vi "myRIO v1.0 Build MUX Configuration DIO.vi"(11 "DIO Channel List":T4) -> (2 "Configuration Bitmask Array":bool[][](array[boolean]), 3 "Channel Reservation List":T1)   [LabVIEW 2021]
uses:
  <vilib>/myRIO/Common/Instrument Driver Framework/myRIO v1.0/DIO/typedefs/DIO Channels List.ctl
  <vilib>/myRIO/Common/Instrument Driver Framework/myRIO v1.0/DIO/typedefs/DIO Channels Enum.ctl
  <vilib>/myRIO/Common/Instrument Driver Framework/myRIO v1.0/Resource Manager/typedefs/myRIO v1.0 Channel Reservation List.ctl
  <vilib>/myRIO/Common/Instrument Driver Framework/myRIO v1.0/Resource Manager/typedefs/myRIO v1.0 Channel Reservation Info.ctl
  <vilib>/myRIO/Common/Instrument Driver Framework/myRIO v1.0/Resource Manager/typedefs/myRIO v1.0 Connector List.ctl
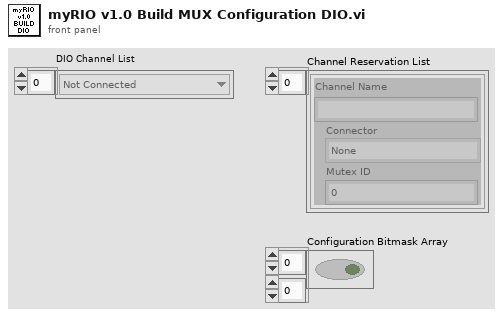
[diagram p1: front panel]
types:
  T1 = typedef "myRIO v1.0 Channel Reservation List.ctl" = T2[]
  T2 = typedef "myRIO v1.0 Channel Reservation Info.ctl" = cluster{"Channel Name":string, "Connector":T3, "Mutex ID":i32}
  T3 = typedef "myRIO v1.0 Connector List.ctl" = enum32{"None", "ConnectorA", "ConnectorB", "ConnectorC"}
  T4 = typedef "DIO Channels List.ctl" = T5[]
  T5 = typedef "DIO Channels Enum.ctl" = enum16{"Not Connected", "C/DIO0", "C/DIO1", "C/DIO2", "C/DIO3", "C/DIO4", "C/DIO5", "C/DIO6", "C/DIO7", "A/DIO0", "A/DIO1", "A/DIO2", "A/DIO3", "A/DIO4", "A/DIO5", "A/DIO6", "A/DIO7", "A/DIO8", "A/DIO9", "A/DIO10", "A/DIO11", "A/DIO12", "A/DIO13", "A/DIO14", "A/DIO15", "A/DIO16", "A/DIO17", "A/DIO18", "A/DIO19", "B/DIO0", "B/DIO1", "B/DIO2", "B/DIO3", "B/DIO4", "B/DIO5", "B/DIO6", "B/DIO7", "B/DIO8", "B/DIO9", "B/DIO10", "B/DIO11", "B/DIO12", "B/DIO13", "B/DIO14", "B/DIO15", "B/DIO16", "B/DIO17", "B/DIO18", "B/DIO19", "LED0", "LED1", "LED2", "LED3", "Button0", "DIO/DIO0", "DIO/DIO1", "DIO/DIO2", "DIO/DIO3", "DIO/DIO4", "DIO/DIO5", "DIO/DIO6", "DIO/DIO7", "DIO/DIO8", "DIO/DIO9", "SPI/CS0", "SPI/CS1", "SPI/CS2", "SPI/CS3", "LED RADIO (Green)", "LED RADIO (Red)", "LED COMM (Green)", "LED COMM (Red)", "LED MODE (Green)", "LED MODE (Red)"}
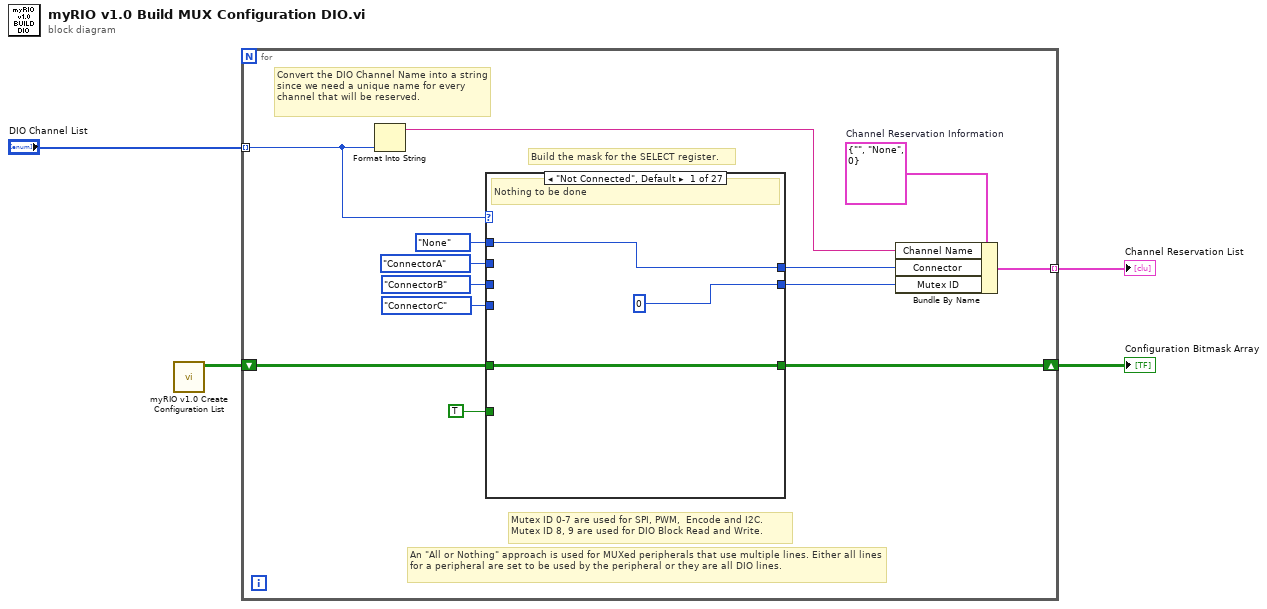
[diagram p0: block diagram]
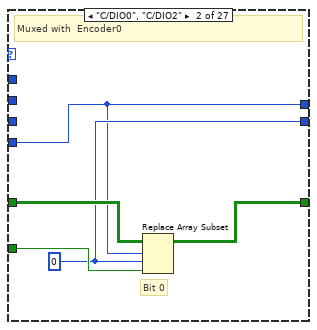
[diagram p2: hidden frame]
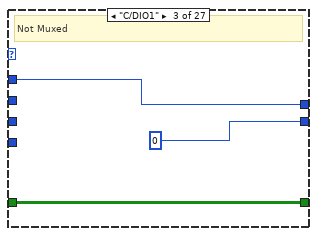
[diagram p3: hidden frame]
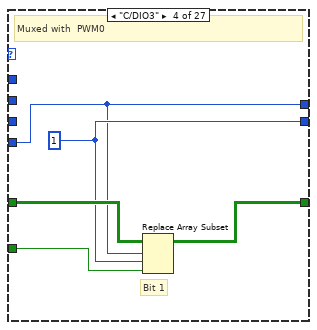
[diagram p4: hidden frame]
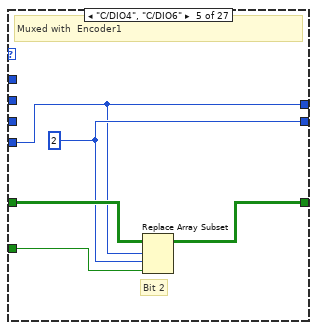
[diagram p5: hidden frame]
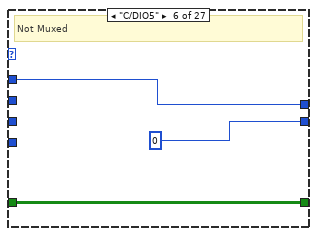
[diagram p6: hidden frame]
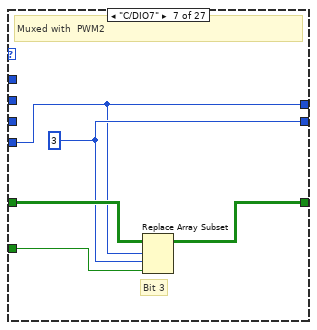
[diagram p7: hidden frame]
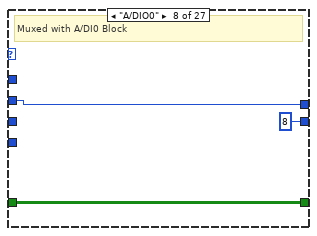
[diagram p8: hidden frame]
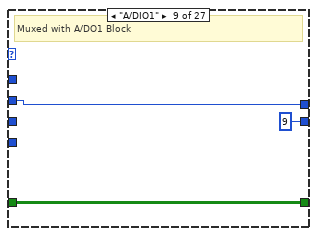
[diagram p9: hidden frame]
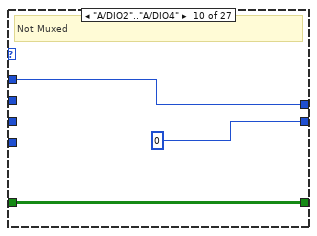
[diagram p10: hidden frame]
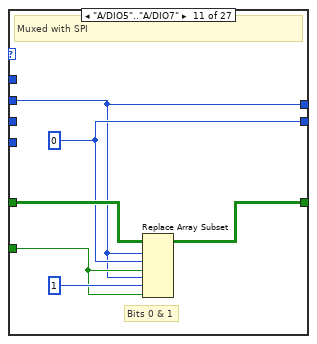
[diagram p11: hidden frame]
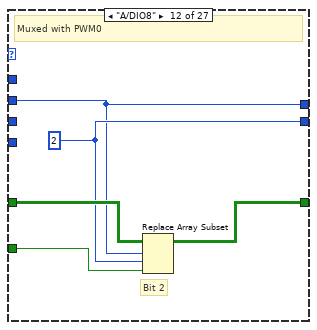
[diagram p12: hidden frame]
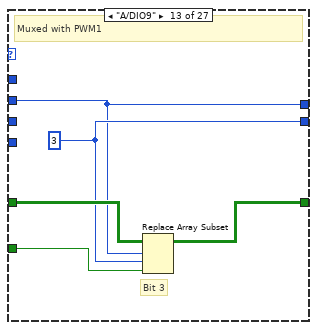
[diagram p13: hidden frame]
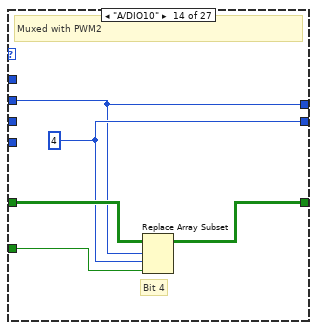
[diagram p14: hidden frame]
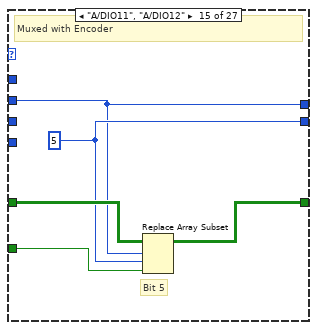
[diagram p15: hidden frame]
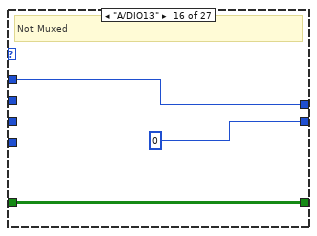
[diagram p16: hidden frame]
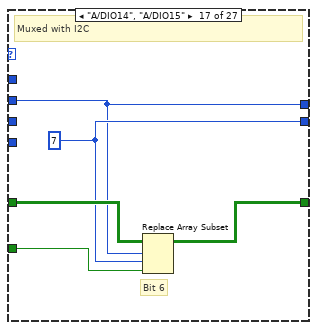
[diagram p17: hidden frame]
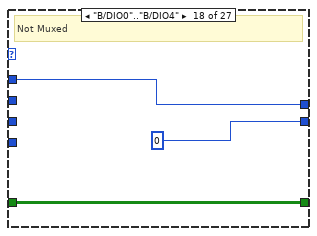
[diagram p18: hidden frame]
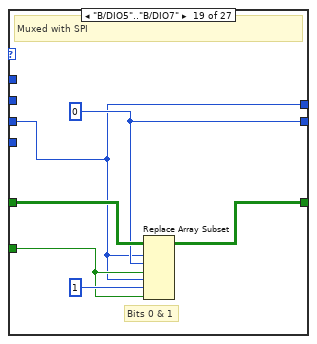
[diagram p19: hidden frame]
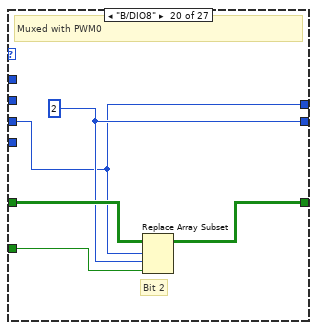
[diagram p20: hidden frame]
diagram:
  n1 = call <vilib>:"myRIO v1.0 Create Configuration List.vi"() -> ("Bitmask Array"=w4:bool[][])  [unwired: 11 in]
  n2 = for {
    shift-right: [w11] -> w3
    shift-left: w4 -> [w12]
    tunnel: "DIO Channel List" -> [w6] mode=indexing
    tunnel: [w7] -> w1 mode=indexing
    w10 = T2 {"Channel Name"="", "Connector"=enum."None", "Mutex ID"=0}  # Channel Reservation Information
    # "Mutex ID 0-7 are used for SPI, PWM,  Encode and I2C.\nMutex ID 8, 9 are used for DIO Block Read and Write."
    # "Convert the DIO Channel Name into a string since we need a unique name for every channel that will be reserved."
    # "An \"All or Nothing\" approach is used for MUXed peripherals that use multiple lines. Either all lines for a peripheral are set to be used by the peripheral or they are all DIO lines."
    # "Build the mask for the SELECT register."
    n3 = Format Into String(w6) -> (resulting string=w5:string)  [unwired: 3 in, 1 out]
    n4 = case shown="\"Not Connected\", Default" w6 {
      tunnel: w12 -> [w20 w25 w28 w33 w38 w41 w46 w47 w50 w55 w61 w66 w71 w76 w81 w84 w89 w92 w97 w103 w108 w113 w118 w121 w126 w129 w132]
      tunnel: [w20 w24 w28 w32 w37 w41 w45 w47 w50 w55 w60 w65 w70 w75 w80 w84 w88 w92 w98 w102 w107 w112 w117 w121 w125 w129 w132] -> w11
      tunnel: myRIO_v1.0_Connector_List."None" ("Connector List") -> [w19 _ w26 _ _ w39 _ _ _ w54 _ _ _ _ _ w82 _ w91 _ _ _ _ _ w119 _ w127 w130]
      tunnel: myRIO_v1.0_Connector_List."ConnectorA" ("Connector List") -> [_ _ _ _ _ _ _ w49 w52 _ w56 w62 w67 w72 w77 _ w85 _ _ _ _ _ _ _ _ _ _]
      tunnel: TRUE ("new element/subarray") -> [_ w23 _ w31 w36 _ w44 _ _ _ w58 w64 w69 w74 w79 _ w87 _ w95 w101 w106 w111 w116 _ w124 _ _]
      tunnel: myRIO_v1.0_Connector_List."ConnectorB" ("Connector List") -> [_ _ _ _ _ _ _ _ _ _ _ _ _ _ _ _ _ _ w93 w99 w104 w109 w114 _ w122 _ _]
      tunnel: myRIO_v1.0_Connector_List."ConnectorC" ("Connector List") -> [_ w21 _ w29 w34 _ w42 _ _ _ _ _ _ _ _ _ _ _ _ _ _ _ _ _ _ _ _]
      tunnel: [0 ("index") w22 0 ("index") w30 w35 0 ("index") w43 8 ("index") 9 ("index") 0 ("index") w57 w63 w68 w73 w78 0 ("index") w86 0 ("index") w94 w100 w105 w110 w115 0 ("index") w123 0 ("index") 0 ("index")] -> w8
      tunnel: [w19 w21 w26 w29 w34 w39 w42 w49 w52 w54 w56 w62 w67 w72 w77 w82 w85 w91 w93 w99 w104 w109 w114 w119 w122 w127 w130] -> w9
      frame "Not Connected", Default {
        # "Nothing to be done"
      }
      frame "C/DIO0", "C/DIO2" {
        w22 = 0 ("index")
        # "Bit 0"
        # "Muxed with  Encoder0"
        n5 = Replace Array Subset(array=w25, new element=w23, index (row)=w21, index (col)=w22) -> (w24:bool[][])
      }
      frame "C/DIO1" {
        # "Not Muxed"
      }
      frame "C/DIO3" {
        w30 = 1 ("index")
        # "Bit 1"
        # "Muxed with  PWM0"
        n6 = Replace Array Subset(array=w33, new element=w31, index (row)=w29, index (col)=w30) -> (w32:bool[][])
      }
      frame "C/DIO4", "C/DIO6" {
        w35 = 2 ("index")
        # "Bit 2"
        # "Muxed with  Encoder1"
        n7 = Replace Array Subset(array=w38, new element=w36, index (row)=w34, index (col)=w35) -> (w37:bool[][])
      }
      frame "C/DIO5" {
        # "Not Muxed"
      }
      frame "C/DIO7" {
        w43 = 3 ("index")
        # "Bit 3"
        # "Muxed with  PWM2"
        n8 = Replace Array Subset(array=w46, new element=w44, index (row)=w42, index (col)=w43) -> (w45:bool[][])
      }
      frame "A/DIO0" {
        # "Muxed with A/DI0 Block"
      }
      frame "A/DIO1" {
        # "Muxed with A/DO1 Block"
      }
      frame "A/DIO2".."A/DIO4" {
        # "Not Muxed"
      }
      frame "A/DIO5".."A/DIO7" {
        w57 = 0 ("index")
        # "Bits 0 & 1"
        # "Muxed with SPI"
        n9 = Replace Array Subset(array=w61, new element #1=w58, index (row) #1=w56, index (col) #1=w57, new element #2=w58, index (row) #2=w56, index (col) #2=1 ("disabled index (col)")) -> (w60:bool[][])
      }
      frame "A/DIO8" {
        w63 = 2 ("index")
        # "Bit 2"
        # "Muxed with PWM0"
        n10 = Replace Array Subset(array=w66, new element=w64, index (row)=w62, index (col)=w63) -> (w65:bool[][])
      }
      frame "A/DIO9" {
        w68 = 3 ("index")
        # "Bit 3"
        # "Muxed with PWM1"
        n11 = Replace Array Subset(array=w71, new element=w69, index (row)=w67, index (col)=w68) -> (w70:bool[][])
      }
      frame "A/DIO10" {
        w73 = 4 ("index")
        # "Bit 4"
        # "Muxed with PWM2"
        n12 = Replace Array Subset(array=w76, new element=w74, index (row)=w72, index (col)=w73) -> (w75:bool[][])
      }
      frame "A/DIO11", "A/DIO12" {
        w78 = 5 ("index")
        # "Bit 5"
        # "Muxed with Encoder"
        n13 = Replace Array Subset(array=w81, new element=w79, index (row)=w77, index (col)=w78) -> (w80:bool[][])
      }
      frame "A/DIO13" {
        # "Not Muxed"
      }
      frame "A/DIO14", "A/DIO15" {
        w86 = 7 ("index")
        # "Bit 6"
        # "Muxed with I2C"
        n14 = Replace Array Subset(array=w89, new element=w87, index (row)=w85, index (col)=w86) -> (w88:bool[][])
      }
      frame "B/DIO0".."B/DIO4" {
        # "Not Muxed"
      }
      frame "B/DIO5".."B/DIO7" {
        w94 = 0 ("index")
        # "Bits 0 & 1"
        # "Muxed with SPI"
        n15 = Replace Array Subset(array=w97, new element #1=w95, index (row) #1=w93, index (col) #1=w94, new element #2=w95, index (row) #2=w93, index (col) #2=1 ("disabled index (col)")) -> (w98:bool[][])
      }
      frame "B/DIO8" {
        w100 = 2 ("index")
        # "Bit 2"
        # "Muxed with PWM0"
        n16 = Replace Array Subset(array=w103, new element=w101, index (row)=w99, index (col)=w100) -> (w102:bool[][])
      }
      frame "B/DIO9" {
        w105 = 3 ("index")
        # "Bit 3"
        # "Muxed with PWM1"
        n17 = Replace Array Subset(array=w108, new element=w106, index (row)=w104, index (col)=w105) -> (w107:bool[][])
      }
      frame "B/DIO10" {
        w110 = 4 ("index")
        # "Bit 4"
        # "Muxed with PWM2"
        n18 = Replace Array Subset(array=w113, new element=w111, index (row)=w109, index (col)=w110) -> (w112:bool[][])
      }
      frame "B/DIO11", "B/DIO12" {
        w115 = 5 ("index")
        # "Bit 5"
        # "Muxed with Encoder"
        n19 = Replace Array Subset(array=w118, new element=w116, index (row)=w114, index (col)=w115) -> (w117:bool[][])
      }
      frame "B/DIO13" {
        # "Not Muxed"
      }
      frame "B/DIO14", "B/DIO15" {
        w123 = 7 ("index")
        # "Bit 6"
        # "Muxed with I2C"
        n20 = Replace Array Subset(array=w126, new element=w124, index (row)=w122, index (col)=w123) -> (w125:bool[][])
      }
      frame "LED0".."LED3" {
        # "Not Muxed"
      }
      frame "Button0" {
        # "Not Muxed"
      }
    }
    n21 = Bundle By Name(cluster=w10, "Channel Name"=w5, "Connector"=w9, "Mutex ID"=w8) -> (w7:T2)
  }
  "Configuration Bitmask Array" <- w3
  "Channel Reservation List" <- w1
